vi "TestGetControlInfo.vi"() -> ()   [LabVIEW 2020]
uses:
  <resource>/Framework/Providers/Open_GDS/ClassProviders/Common/CommonVIs/CommonVIs_AttributeInfoType.ctl
  <resource>/Framework/Providers/Open_GDS/ClassProviders/Common/CommonVIs/CommonVIs_AttributeDataType.ctl
  <resource>/Framework/Providers/Open_GDS/ClassProviders/Common/CommonVIs/CommonVIs_VisibilityType.ctl
panel:
  out "Array 2":T1[](array[typedef])
  in  "File Path":refnum<class>[](array[class])
  out "Array":T1[](array[typedef])
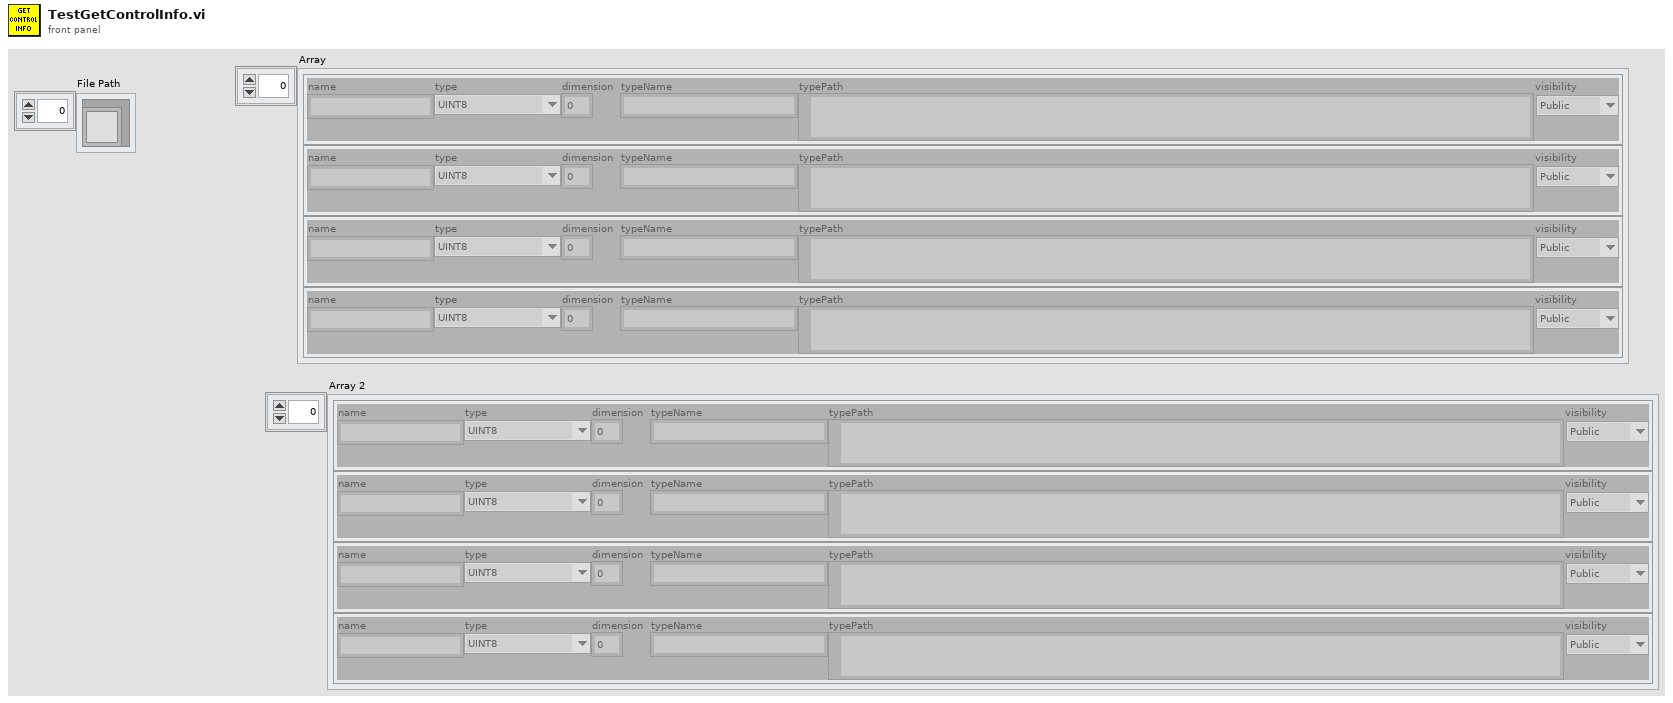
[diagram p1: front panel]
types:
  T1 = typedef "CommonVIs_AttributeInfoType.ctl" = cluster{"name":string, "type":T2, "dimension":i32, "typeName":string, "typePath":path, "visibility":T3}
  T2 = typedef "CommonVIs_AttributeDataType.ctl" = enum16{"UINT8", "INT8", "UINT16", "INT16", "UINT32", "INT32", "UINT64", "INT64", "SGL", "DBL", "EXT", "CSG", "CDB", "CXT", "TimeStamp", "STRING", "PATH", "BOOL", "ENUM", "RefNum", "VIRefNum", "LabVIEW Class", "Cluster", "Variant", "TypeDef", "Waveform", "LabVIEW Object", "Other", "void", "Set", "Map"}
  T3 = typedef "CommonVIs_VisibilityType.ctl" = enum16{"Public", "Private", "Protected"}
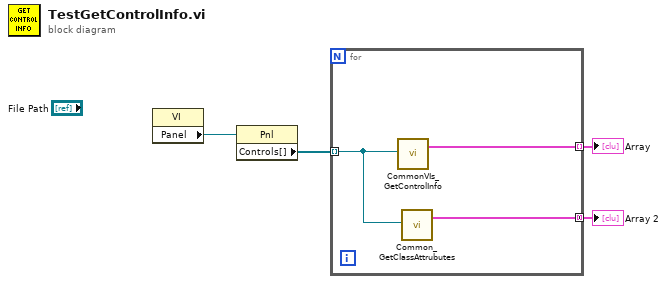
[diagram p0: block diagram]
diagram:
  n1 = property class="VI"() -> ("Panel"=w4:refnum<vi>)  [unwired: 2 in, 2 out]
  n2 = property class="Pnl"(reference=w4) -> ("Controls[]"=w3:refnum<vi>[])  [unwired: 1 in, 2 out]
  n3 = for {
    tunnel: w3 -> [w6] mode=indexing
    tunnel: [w7] -> w2 mode=indexing
    tunnel: [w5] -> w1 mode=concatenating
    n4 = call <resource>:"CommonVIs_GetControlInfo.vi"("CtlRefnum"=w6) -> ("attributeInfoType"=w7:T1)  [unwired: 17 in, 1 out]
    n5 = call <resource>:"Common_GetClassAttrubutes.vi"("CtlRefnum"=w6) -> ("attributeInfo"=w5:T1[])  [unwired: 16 in, 2 out]
  }
  "Array" <- w2
  "Array 2" <- w1
